vi "AM-sinal-modulation.vi"() -> ()   [LabVIEW 2013]
panel:
  in  "N":dbl=1.0 caption="Numero de ciclos" format="%#_13g"
  out "mod":cluster{i32[], dbl[]}(graph) caption="Modulação"
  out "Portadora":cluster{i32[], dbl[]}(graph)
  out "Informação":cluster{i32[], dbl[]}(graph)
  in  "K":dbl
  in  "Nc":dbl caption="Numero de amostras"
  in  "fm":dbl caption="Frequencia do sinal modulador"
  in  "fp":dbl caption="Frequencia da portadora"
  in  "E0":dbl caption="Amplitude da portadora"
  in  "Em":dbl caption="Amplitude do sinal modulador"
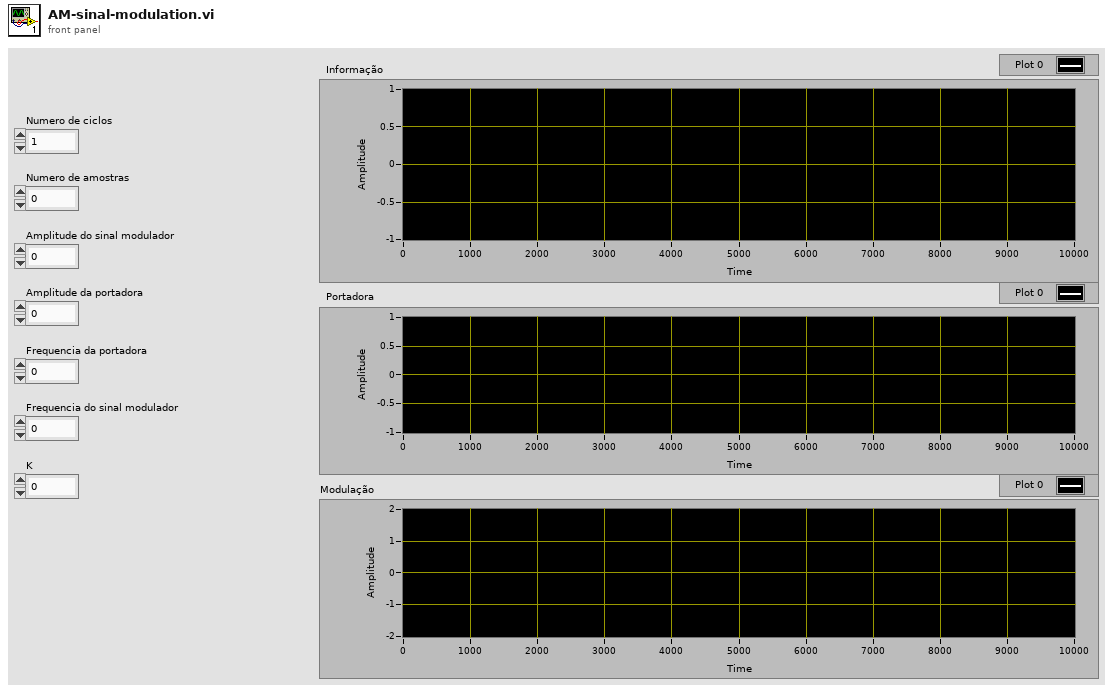
[diagram p1: front panel]
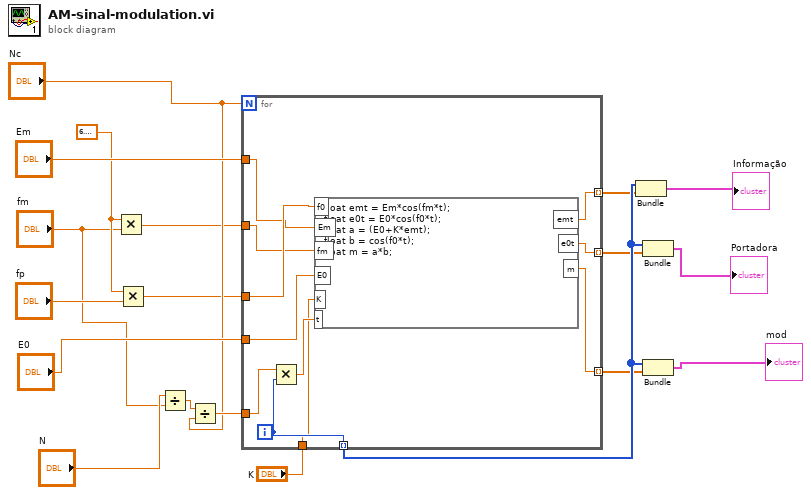
[diagram p0: block diagram]
diagram:
  w18 = 6.283185307179586
  n1 = Multiply(x=w18, y="fm") -> (x*y=w10:dbl)
  n2 = Multiply(x=w18, y="fp") -> (x*y=w11:dbl)
  n3 = Divide(x="N", y="fm") -> (x/y=w14:dbl)
  n4 = Divide(x=w14, y="Nc") -> (x/y=w13:dbl)
  n5 = for {
    N: "Nc" -> [_]
    tunnel: "Em" -> [w23]
    tunnel: "E0" -> [w24]
    tunnel: w10 -> [w25]
    tunnel: w11 -> [w26]
    tunnel: [w29] -> w7 mode=indexing
    tunnel: w13 -> [w30]
    tunnel: "K" -> [w27]
    tunnel: [w22] -> w6 mode=indexing
    tunnel: [w21] -> w5 mode=indexing
    tunnel: [w20] -> w4 mode=indexing
    i -> [w29]
    n6 = Multiply(x=w30, y=w29) -> (x*y=w28:dbl)
    n7 = formula code="float emt = Em*cos(fm*t);\nfloat e0t = E0*cos(f0*t);\nfloat a = (E0+K*emt);\nfloat b = cos(f0*t);\nfloat m = a*b;"("fm"=w25, "f0"=w26, "Em"=w23, "E0"=w24, "t"=w28, "K"=w27) -> ("emt"=w22:dbl, "e0t"=w21:dbl, "m"=w20:dbl)
  }
  n8 = Bundle(w7, w6) -> (→"Informação":cluster{i32[], dbl[]})  [unwired: 1 in]
  n9 = Bundle(w7, w5) -> (→"Portadora":cluster{i32[], dbl[]})  [unwired: 1 in]
  n10 = Bundle(w7, w4) -> (→"mod":cluster{i32[], dbl[]})  [unwired: 1 in]
